vi "Read Minor Grid Color.vi"(4 "error in (no error)":errorcluster, 6 "Container State":T4, 7 "Display State In":T1={"Graph Visible Items"={"Plot Legend"=FALSE, "Scale Legend"=FALSE, "Graph Palette"=FALSE, "Cursor Legend"=FALSE, "X Scrollbar"=FALSE}, "View Table"=FALSE, "Table Visible Items"={"Vertical Scrollbar"=FALSE, "Horizontal Scrollbar"=FALSE, "Row Headers"=FALSE, "Column Headers"=FALSE, "Vertical Lines"=FALSE, "Horizontal Lines"=FALSE}, "Header Font"={"Font Name"="", "Size"=0, "Bold"=FALSE, "Italic"=FALSE, "Underline"=FALSE, "Strikeout"=FALSE, "Color"=0}, "Cell Font"={"Font Name"="", "Size"=0, "Bold"=FALSE, "Italic"=FALSE, "Underline"=FALSE, "Strikeout"=FALSE, "Color"=0}, "Description and Tip..."={"Description"="", "Tip"=""}, "Moveable Splitter Position"=0, "Measurement Cursor Configuration"={"relative to t0"={"enable relative time"=FALSE, "Relative times (DT)"=[], "color"=0}, "range"={"enable range"=FALSE, "T1"=0.0, "T2"=0.0, "Fixed interval (T2-T1)"=0.0, "T1 color"=0, "T2 color"=0, "enable shading"=FALSE}, "periodic"={"enable periodic"=FALSE, "First event (E1)"=0.0, "Number events (Ei)"=0, "Event spacing (s)"=0.0, "First color"=0, "Events color"=0}, "absolute timestamp"={"enable absolute"=FALSE, "Timestamps (TS)"=[], "color"=0}}, "X Increment"=0.0, "X Scale"={"Label Visible"=FALSE, "Label Text"="Time (s)", "Time Mode"=enum."Relative", "Format String"=""}, "Y Scale"={"Label Visible"=FALSE, "Label Text"="", "Scaling"=enum."Engineering Units", "Format String"=""}, "Colors"={"background"=16777215, "major grid"=8355711, "minor grid"=16777226, "font"=0}, "Cursors"={"List"=[], "Tags"=[]}, "Plots"=[], "Plot Color Wheel"=[3381759, 32768, 982784, 4375295, 13827953, 13457919, 16757522, 4343295, 16728758, 12095254], "registered user events"=variant}) -> (0 "error out":errorcluster, 2 "Value":u32(colorbox), 3 "Display State Out":T1={"Graph Visible Items"={"Plot Legend"=FALSE, "Scale Legend"=FALSE, "Graph Palette"=FALSE, "Cursor Legend"=FALSE, "X Scrollbar"=FALSE}, "View Table"=FALSE, "Table Visible Items"={"Vertical Scrollbar"=FALSE, "Horizontal Scrollbar"=FALSE, "Row Headers"=FALSE, "Column Headers"=FALSE, "Vertical Lines"=FALSE, "Horizontal Lines"=FALSE}, "Header Font"={"Font Name"="", "Size"=0, "Bold"=FALSE, "Italic"=FALSE, "Underline"=FALSE, "Strikeout"=FALSE, "Color"=0}, "Cell Font"={"Font Name"="", "Size"=0, "Bold"=FALSE, "Italic"=FALSE, "Underline"=FALSE, "Strikeout"=FALSE, "Color"=0}, "Description and Tip..."={"Description"="", "Tip"=""}, "Moveable Splitter Position"=0, "Measurement Cursor Configuration"={"relative to t0"={"enable relative time"=FALSE, "Relative times (DT)"=[], "color"=0}, "range"={"enable range"=FALSE, "T1"=0.0, "T2"=0.0, "Fixed interval (T2-T1)"=0.0, "T1 color"=0, "T2 color"=0, "enable shading"=FALSE}, "periodic"={"enable periodic"=FALSE, "First event (E1)"=0.0, "Number events (Ei)"=0, "Event spacing (s)"=0.0, "First color"=0, "Events color"=0}, "absolute timestamp"={"enable absolute"=FALSE, "Timestamps (TS)"=[], "color"=0}}, "X Increment"=0.0, "X Scale"={"Label Visible"=FALSE, "Label Text"="Time (s)", "Time Mode"=enum."Relative", "Format String"=""}, "Y Scale"={"Label Visible"=FALSE, "Label Text"="", "Scaling"=enum."Engineering Units", "Format String"=""}, "Colors"={"background"=16777215, "major grid"=8355711, "minor grid"=16777226, "font"=0}, "Cursors"={"List"=[], "Tags"=[]}, "Plots"=[], "Plot Color Wheel"=[3381759, 32768, 982784, 4375295, 13827953, 13457919, 16757522, 4343295, 16728758, 12095254], "registered user events"=variant})   [LabVIEW 2017, in "Waveforms with Cursors.xctl"]
uses:
  <vilib>/addons/_XControls/Waveforms with Cursors/Waveforms with Cursors.xctl
  <vilib>/_xctls/Container State.ctl
  <vilib>/addons/_XControls/Waveforms with Cursors/Controls/State.ctl
  <vilib>/Utility/miscctls.llb/LVFontTypeDef.ctl
  <vilib>/addons/_XControls/Waveforms with Cursors/Controls/Waveform Cursor Configuration.ctl
  <vilib>/_xctls/XControlSupport.lvlib
panel:
  # "Replace the Value Indicator below with an Indicator of desired type.\nDo not remove this Indicator or the others from the connector pane. \nDo not change the connector pane pattern.\nThe Value Indicator should always be the second terminal from top on the output side in the connector pane."
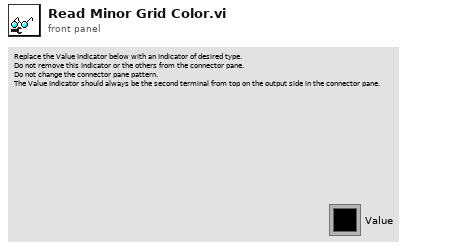
[diagram p1: front panel]
types:
  T1 = typedef "Waveforms with Cursors.xctl/State.ctl" = cluster{"Graph Visible Items":cluster{"Plot Legend":bool, "Scale Legend":bool, "Graph Palette":bool, "Cursor Legend":bool, "X Scrollbar":bool}, "View Table":bool, "Table Visible Items":cluster{"Vertical Scrollbar":bool, "Horizontal Scrollbar":bool, "Row Headers":bool, "Column Headers":bool, "Vertical Lines":bool, "Horizontal Lines":bool}, "Header Font":T2, "Cell Font":T2, "Description and Tip...":cluster{"Description":string, "Tip":string}, "Moveable Splitter Position":i32, "Measurement Cursor Configuration":T3, "X Increment":dbl, "X Scale":cluster{"Label Visible":bool, "Label Text":string, "Time Mode":enum16{"Relative", "Absolute"}, "Format String":string}, "Y Scale":cluster{"Label Visible":bool, "Label Text":string, "Scaling":enum16{"Engineering Units", "Voltage"}, "Format String":string}, "Colors":cluster{"background":u32, "major grid":u32, "minor grid":u32, "font":u32}, "Cursors":cluster{"List":cluster{"Name":string, "Color":u32, "Style":i32, "Point Style":u8, "Name Visible":bool, "Allow Drag":bool, "Cursor Mode":u32, "Plot":i32, "Index":i32, "Position":cluster{"X":dbl, "Y":dbl}, "X Scale":u32, "Y Scale":u32, "Watch Plots":i32[], "Watch All Plots":bool, "Plot Area":i32, "Label Offset":cluster{"X":dbl, "Y":dbl}}[], "Tags":variant[]}, "Plots":cluster{"Name":string, "Line Color":u32, "Line Style":u8, "Line Width":u8, "Fill/Point Color":u32, "Point Style":u8, "Fill To":i16, "Interpolation":u8, "Anti-aliased":bool}[], "Plot Color Wheel":u32[], "registered user events":variant}
  T2 = typedef "LVFontTypeDef.ctl" = cluster{"Font Name":string, "Size":u16, "Bold":bool, "Italic":bool, "Underline":bool, "Strikeout":bool, "Color":u32}
  T3 = typedef "Waveforms with Cursors.xctl/Waveform Cursor Configuration.ctl" = cluster{"relative to t0":cluster{"enable relative time":bool, "Relative times (DT)":dbl[], "color":u32}, "range":cluster{"enable range":bool, "T1":dbl, "T2":dbl, "Fixed interval (T2-T1)":dbl, "T1 color":u32, "T2 color":u32, "enable shading":bool}, "periodic":cluster{"enable periodic":bool, "First event (E1)":dbl, "Number events (Ei)":i32, "Event spacing (s)":dbl, "First color":u32, "Events color":u32}, "absolute timestamp":cluster{"enable absolute":bool, "Timestamps (TS)":timestamp[], "color":u32}}
  T4 = typedef "XControlSupport.lvlib/Container State.ctl" = cluster{"Indicator?":bool, "Run Mode?":bool, " Refnum":refnum<vi>}
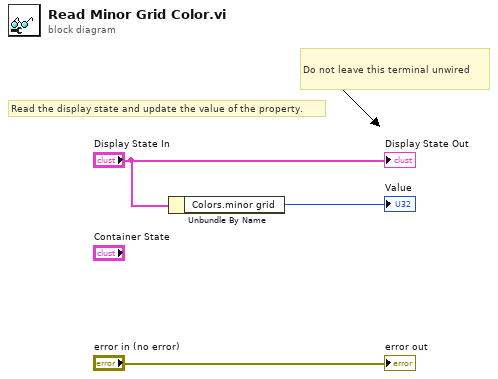
[diagram p0: block diagram]
diagram:
  # "Do not leave this terminal unwired"
  # "Read the display state and update the value of the property."
  n1 = Unbundle By Name("Display State In") -> ("Colors.minor grid"=→"Value":u32)
  "error out" <- "error in (no error)"
  "Display State Out" <- "Display State In"
